vi "Read Field (U16).vi"(7 "field name":string, 8 "error in (no error)":errorcluster, 10 "default":u16, 11 "PV Data in":refnum<class "PV Data.lvclass">) -> (0 "error out":errorcluster, 2 "value":u16, 3 "PV Data out":refnum<class "PV Data.lvclass">)   [LabVIEW 2020, in "PV Access.lvlib" / "PV Data.lvlib" / "PV Data.lvclass"]
uses:
  PV Data.lvclass
  PV Data.lvclass/PV Data.ctl
  PV Access.lvlib
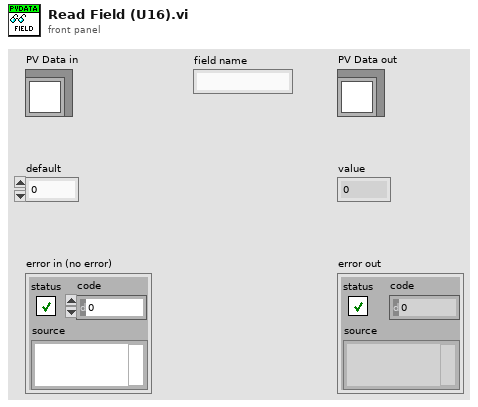
[diagram p1: front panel]
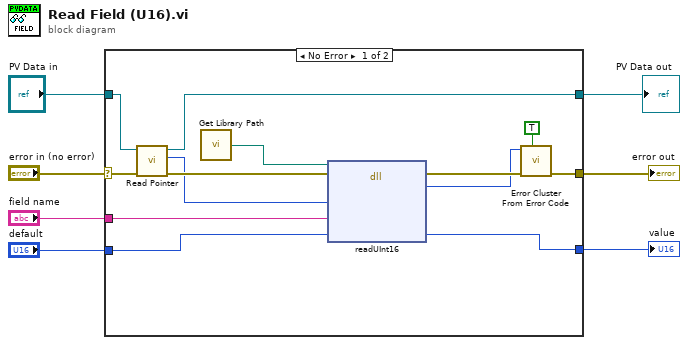
[diagram p0: block diagram]
diagram:
  n1 = case shown="No Error" "error in (no error)" {
    selector: "error in (no error)" -> [w13 w23]
    tunnel: [w14 w23] -> w7
    tunnel: "PV Data in" -> [w11 w22]
    tunnel: [w9 w22] -> w2
    tunnel: "default" -> [w20 w21]
    tunnel: [w19 w21] -> w4
    tunnel: "field name" -> [w8 _]
    frame No Error {
      n2 = call-dynamic "Read Pointer.vi"("error in (no error)"=w13, "Pointer Base in"=w11) -> ("error out"=w12:errorcluster, "Pointer"=w10:i64, "Pointer Base out"=w9:refnum<class "PV Data.lvclass">)  [unwired: 7 in]
      n3 = call "Get Library Path.vi"() -> ("Path"=w18:path)  [unwired: 1 in]
      n4 = dll-call lib="?" fn="readUInt16"(path in=w18, error in=w12, "value"=w10, "field_name"=w8, "result"=w20) -> (error out=w16:errorcluster, "err_code"=w15:i32, "result"=w19:u16)  [unwired: 3 in, 1 out]
      n5 = call <vilib>:"Error Cluster From Error Code.vi"("show call chain? (False)"=TRUE, "error in (no error)"=w16, "error code (0)"=w15) -> ("error out"=w14:errorcluster)  [unwired: 6 in]
    }
    frame Error {
    }
  }
  "error out" <- w7
  "value" <- w4
  "PV Data out" <- w2
